vi "Initialize Generic Serial Arm.vi"(0 "Robot Arm in":refnum<class "Robot Arm.lvclass">, 5 "kinematic parameters":T4(array[cluster]), 7 "dynamic parameters":T2[](array[typedef]), 9 "Home Transform T0":T1, 11 "error in (no error)":errorcluster) -> (4 "Robot Arm out":refnum<class "Robot Arm.lvclass">, 15 "error out":errorcluster)   [LabVIEW 2013, in "Robot Arm.lvclass"]
uses:
  Robot Arm.lvclass
  <vilib>/robotics/Kinematics/Link/Joint Type.ctl
  <vilib>/robotics/Kinematics/DH Dynamic Parameters.ctl
  <vilib>/Analysis/Matrix/Datatypes/RealMatrix.ctl
  Link/Link.lvclass
  Link/Link.lvclass/Link.ctl
  Robot Arm.lvclass/Robot Arm.ctl
  <vilib>/robotics/Utilities/NI_Robotics Utilities.lvlib
  <vilib>/robotics/Kinematics/Link/NI_Robotics_Link.lvclass
  <vilib>/Analysis/Matrix/NI_Matrix.lvlib
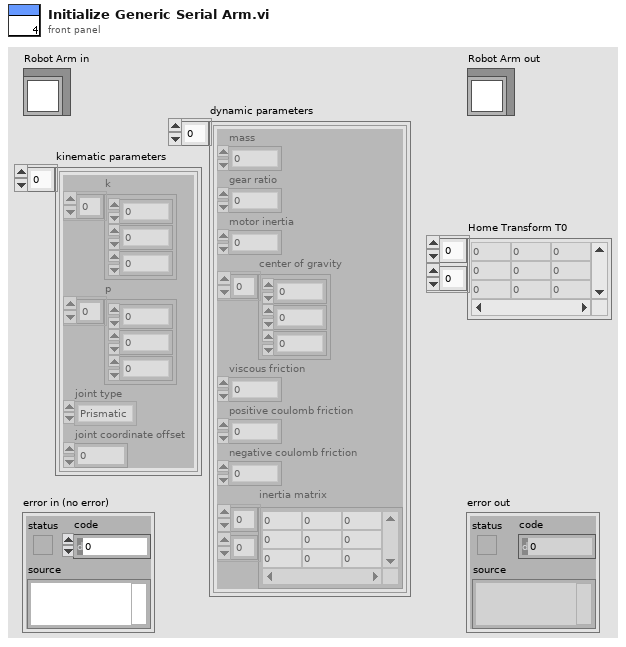
[diagram p1: front panel]
types:
  T1 = typedef "NI_Matrix.lvlib/RealMatrix.ctl" = dbl[][]
  T2 = typedef "DH Dynamic Parameters.ctl" = cluster{"mass":dbl, "gear ratio":dbl, "motor inertia":dbl, "center of gravity":dbl[], "viscous friction":dbl, "positive coulomb friction":dbl, "negative coulomb friction":dbl, "inertia matrix":T1}
  T3 = typedef "NI_Robotics_Link.lvclass/Joint Type.ctl" = enum16{"Revolute", "Prismatic"}
  T4 = cluster{"k":dbl[], "p":dbl[], "joint type":T3, "joint coordinate offset":dbl}[]
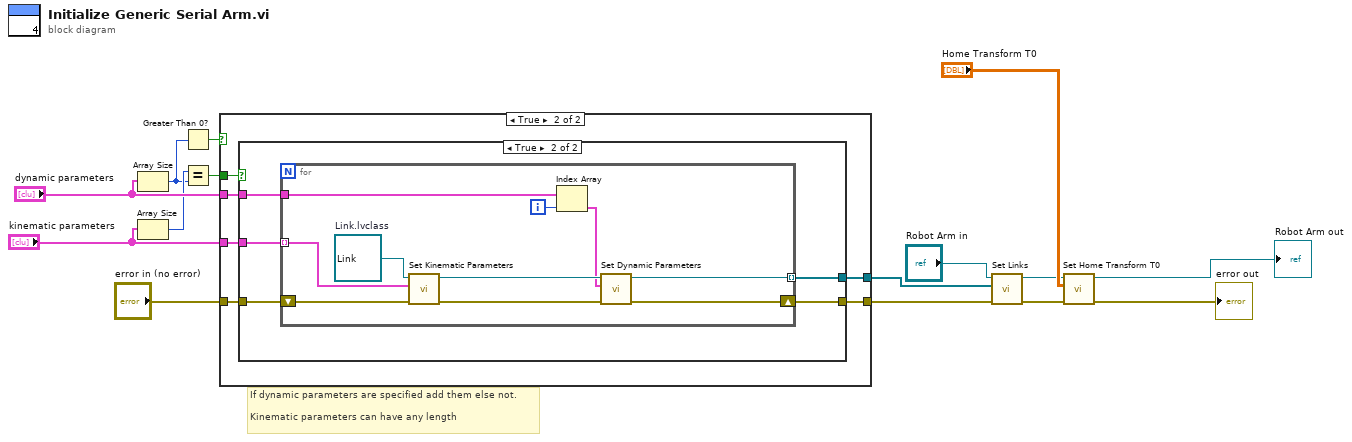
[diagram p0: block diagram]
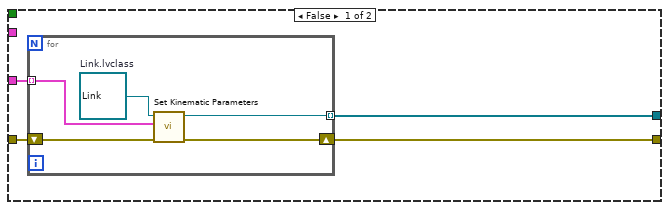
[diagram p2: hidden frame]
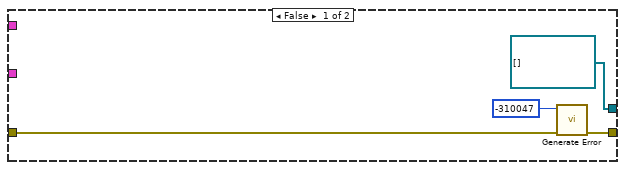
[diagram p3: hidden frame]
diagram:
  # "If dynamic parameters are specified add them else not.\n\nKinematic parameters can have any length"
  n1 = Array Size(array="dynamic parameters") -> (size(s)=w9:i32)
  n2 = Array Size(array="kinematic parameters") -> (size(s)=w10:i32)
  n3 = Greater Than 0?(x=w9) -> (x > 0?=w12:bool)
  n4 = Equal?(x=w10, y=w9) -> (x = y?=w8:bool)
  n5 = case shown="True" w12 {
    tunnel: "kinematic parameters" -> [w19 w30]
    tunnel: "error in (no error)" -> [w18 w29]
    tunnel: [w16 w28] -> w15
    tunnel: [w17 w27] -> w14
    tunnel: "dynamic parameters" -> [_ w26]
    tunnel: w8 -> [_ w25]
    frame False {
      n6 = for {
        tunnel: w19 -> [w24] mode=indexing
        shift-right: [w21] -> w16
        shift-left: w18 -> [w23]
        tunnel: [w22] -> w17 mode=indexing
        w20 = refnum<class "Link.lvclass"> refnum  # Link.lvclass
        n7 = call "Set Kinematic Parameters.vi"("error in (no error)"=w23, "kinematic parameters"=w24, "Link in"=w20) -> ("error out"=w21:errorcluster, "Link out"=w22:refnum<class "Link.lvclass">)  [unwired: 7 in]
      }
    }
    frame True {
      n8 = case shown="True" w25 {
        tunnel: w30 -> [_ w39]
        tunnel: w29 -> [w32 w38]
        tunnel: [w33 w37] -> w28
        tunnel: [refnum<class "Link.lvclass">[] [] w36] -> w27
        tunnel: w26 -> [_ w35]
        frame False {
          n9 = call <vilib>:"Generate Error.vi"("error in (no error)"=w32, "code"=-310047) -> ("error out"=w33:errorcluster)  [unwired: 9 in]
        }
        frame True {
          n10 = for {
            tunnel: w39 -> [w40] mode=indexing
            tunnel: w35 -> [w46]
            tunnel: [w44] -> w36 mode=indexing
            shift-right: [w45] -> w37
            shift-left: w38 -> [w43]
            i -> [w41]
            w49 = refnum<class "Link.lvclass"> refnum  # Link.lvclass
            n11 = call "Set Kinematic Parameters.vi"("error in (no error)"=w43, "kinematic parameters"=w40, "Link in"=w49) -> ("error out"=w47:errorcluster, "Link out"=w48:refnum<class "Link.lvclass">)  [unwired: 7 in]
            n12 = Index Array(array=w46, index=w41) -> (element=w42:T2)
            n13 = call "Set Dynamic Parameters.vi"("error in (no error)"=w47, "dynamic parameters"=w42, "Link in"=w48) -> ("error out"=w45:errorcluster, "Link out"=w44:refnum<class "Link.lvclass">)  [unwired: 7 in]
          }
        }
      }
    }
  }
  n14 = call "Set Links.vi"("error in (no error)"=w15, "Links"=w14, "Robot Arm in"="Robot Arm in") -> ("error out"=w3:errorcluster, "Robot Arm out"=w4:refnum<class "Robot Arm.lvclass">)  [unwired: 7 in]
  n15 = call "Set Home Transform T0.vi"("error in (no error)"=w3, "T0 Transform"="Home Transform T0", "Robot Arm in"=w4) -> ("error out"=→"error out":errorcluster, "Robot Arm out"=→"Robot Arm out":refnum<class "Robot Arm.lvclass">)  [unwired: 7 in]
